vi "Status_read.vi"(8 "error in (no error)":errorcluster, 9 "Combo Box":string(combo), 11 "IT6932A in":refnum<class "IT6932A.lvclass">) -> (0 "error out":errorcluster, 1 "read buffer":string, 3 "IT6932A out":refnum<class "IT6932A.lvclass">)   [LabVIEW 2023, in "IT6932A.lvclass"]
uses:
  IT6932A.lvclass
  IT6932A.lvclass/IT6932A.ctl
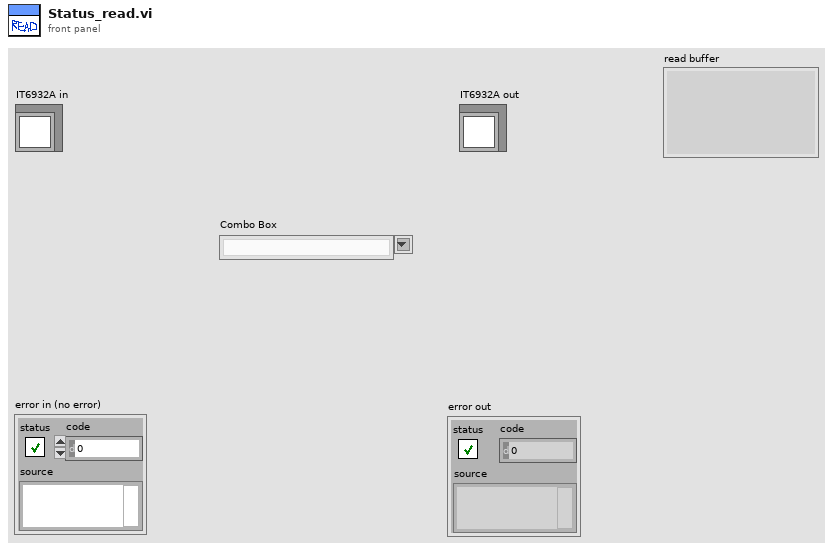
[diagram p1: front panel]
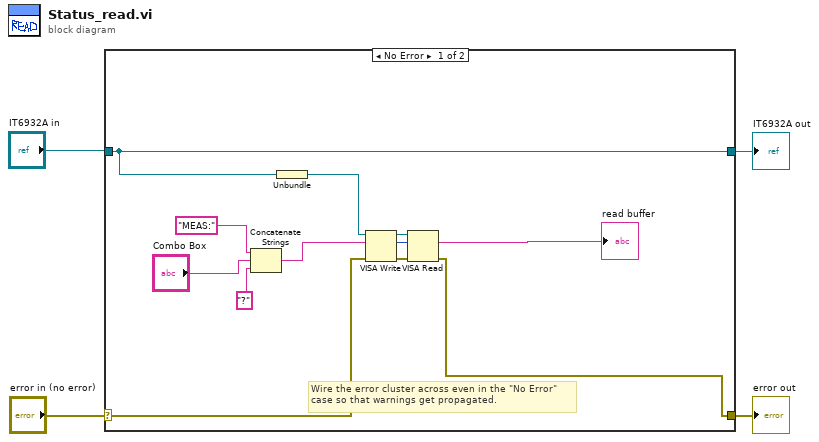
[diagram p0: block diagram]
diagram:
  n1 = case shown="No Error" "error in (no error)" {
    selector: "error in (no error)" -> [w13 w18]
    tunnel: [w11 w18] -> w3
    tunnel: [w9 w17] -> w1
    tunnel: "IT6932A in" -> [w9 w17]
    frame No Error {
      # "Wire the error cluster across even in the \"No Error\"\ncase so that warnings get propagated."
      n2 = Concatenate Strings("MEAS:" ("write buffer"), "Combo Box", "?" ("write buffer")) -> (w5:string)
      n3 = Unbundle(w9) -> (w10:refnum<visa-resource-name>)
      n4 = VISA Write(VISA resource name=w10, write buffer=w5, error in (no error)=w13) -> (VISA resource name out=w16:refnum<visa-resource-name>, return count=w14:u32, error out=w12:errorcluster)
      n5 = VISA Read(VISA resource name=w16, byte count=w14, error in (no error)=w12) -> (read buffer=→"read buffer":string, error out=w11:errorcluster)  [unwired: 2 out]
    }
    frame Error {
    }
  }
  "error out" <- w3
  "IT6932A out" <- w1
